vi "Debug_Convert_Data_to_String.vi"(8 "error in (no error)":errorcluster, 11 "AB_Destination in":refnum<class "AB_Destination.lvclass">) -> (0 "error out":errorcluster, 2 "classData":string, 3 "AB_Destination out":refnum<class "AB_Destination.lvclass">)   [LabVIEW 2020, in "AB_Destination.lvclass"]
uses:
  <vilib>/AppBuilder/AB_Classes/Destination/AB_Destination.lvclass
  <vilib>/AppBuilder/AB_Classes/Destination/AB_Destination.lvclass/AB_Destination.ctl
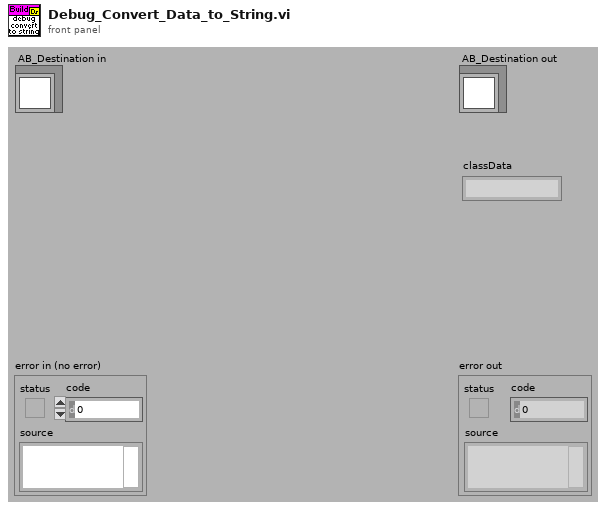
[diagram p1: front panel]
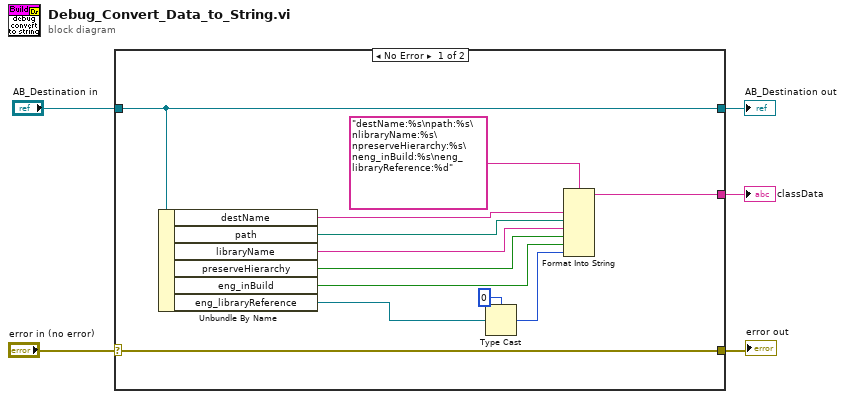
[diagram p0: block diagram]
diagram:
  n1 = case shown="No Error" "error in (no error)" {
    selector: "error in (no error)" -> [w17 w19]
    tunnel: [w17 w19] -> w4
    tunnel: [w16 w18] -> w2
    tunnel: "AB_Destination in" -> [w16 w18]
    tunnel: [w9 _] -> w1
    frame No Error {
      n2 = Unbundle By Name(w16) -> ("destName"=w14:string, "path"=w13:path, "libraryName"=w12:string, "preserveHierarchy"=w6:bool, "eng_inBuild"=w7:bool, "eng_libraryReference"=w11:refnum<vi>)
      n3 = Type Cast(type=u32 0, x=w11) -> (*(type *) &x=w8:u32)
      n4 = Format Into String(format string="destName:%s\npath:%s\nlibraryName:%s\npreserveHierarchy:%s\neng_inBuild:%s\neng_libraryReference:%d", w14, w13, w12, w6, w7, w8) -> (resulting string=w9:string)  [unwired: 2 in, 1 out]
    }
    frame Error {
    }
  }
  "error out" <- w4
  "AB_Destination out" <- w2
  "classData" <- w1
